vi "Read Listened To Msg.vi"(11 "Core Actor in":refnum<class "Core Actor.lvclass">) -> (2 "Listened To Msg":bool)   [LabVIEW 2025, in "jettl.lvlib" / "Core Actor.lvlib" / "Core Actor.lvclass"]
uses:
  Core Actor.lvclass
  Core Actor.lvclass/Core Actor.ctl
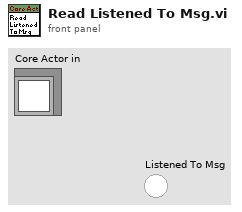
[diagram p1: front panel]
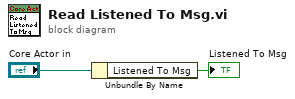
[diagram p0: block diagram]
diagram:
  n1 = Unbundle By Name("Core Actor in") -> ("Listened To Msg"=→"Listened To Msg":bool)
